vi "LVClass_WavefrontCorrector Get Actuator Current Position.vi"(0 "WavefrontCorrector in":refnum<class "WavefrontCorrector.lvclass">, 5 "Index of actuator":i32, 11 "error in (no error)":errorcluster) -> (4 "WavefrontCorrector out":refnum<class "WavefrontCorrector.lvclass">, 6 "Position":i32, 15 "error out":errorcluster)   [LabVIEW 2020, in "WavefrontCorrector.lvclass"]
doc: "Get current position of actuator.\n\n<B>correctorIn</B> : WavefrontCorrector object.\n<B>correctorOut</B> : WavefrontCorrector object.\n<B>actuator_index</B> : Index of the actuator.\n<B>position</B> : Position of the actuator."
uses:
  WavefrontCorrector.lvclass
  WavefrontCorrector.lvclass/WavefrontCorrector.ctl
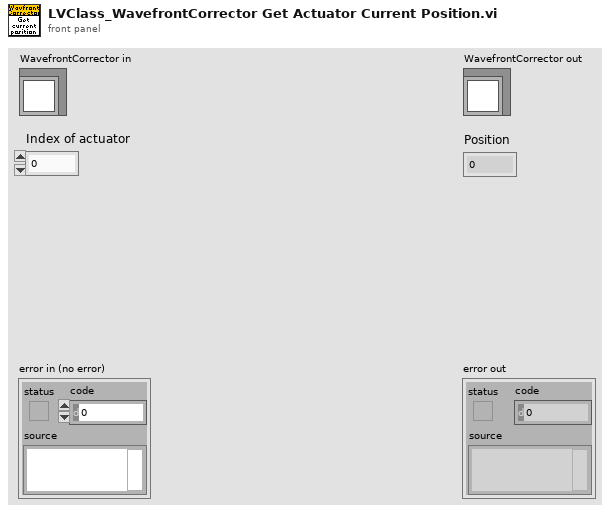
[diagram p1: front panel]
types:
  T1 = typedef "ClassID.ctl" = i64
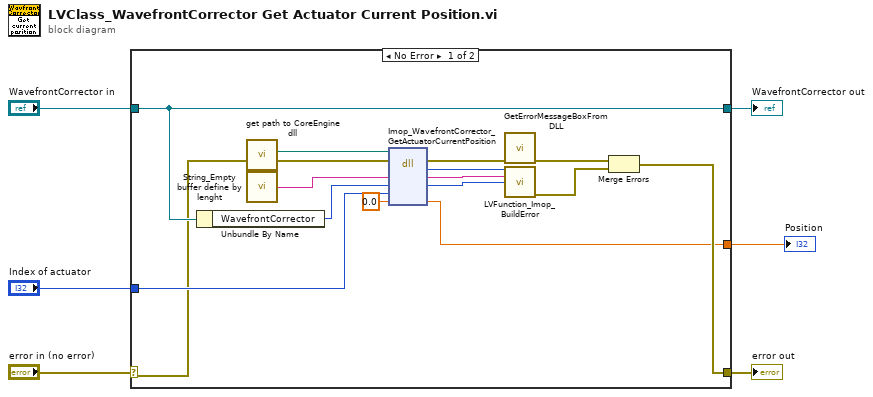
[diagram p0: block diagram]
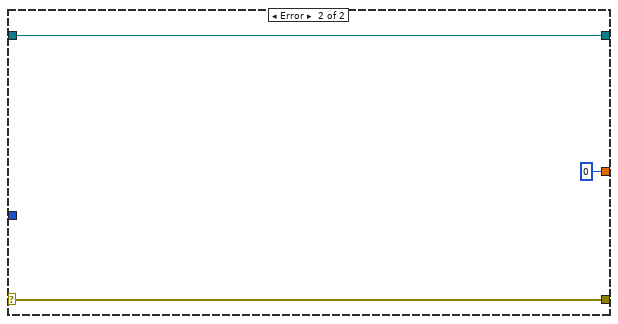
[diagram p2: hidden frame]
diagram:
  n1 = case shown="No Error" "error in (no error)" {
    selector: "error in (no error)" -> [w10 w24]
    tunnel: [w11 w24] -> w5
    tunnel: [w19 w23] -> w3
    tunnel: "WavefrontCorrector in" -> [w19 w23]
    tunnel: "Index of actuator" -> [w17 _]
    tunnel: [w9 0 ("Position")] -> w1
    frame No Error {
      n2 = Unbundle By Name(w19) -> ("WavefrontCorrector"=w18:T1)
      n3 = call "get path to CoreEngine dll.vi"() -> ("path to wavekit library"=w21:path)  [unwired: 14 in, 1 out]
      n4 = call "String_Empty buffer define by lenght.vi"() -> ("Empty buffer"=w20:string)  [unwired: 1 in]
      n5 = dll-call lib="D:/FLE/0.Code/CoreEngine4_Suite/LV2011_interface/DLLs/c_interface_vc100.dll" fn="Imop_WavefrontCorrector_GetActuatorCurrentPosition"(path in=w21, error in=w10, "Message"=w20, "WavefrontCorrector"=w18, "Index of actuator"=w17, "Position"=sgl 0.0) -> (error out=w16:errorcluster, "return type"=w14:i32, "Message"=w13:string, "WavefrontCorrector"=w7:i64, "Position"=w9:sgl)  [unwired: 2 in, 1 out]
      n6 = call "GetErrorMessageBoxFromDLL.vi"("error IN"=w16) -> ("error OUT"=w15:errorcluster)  [unwired: 10 in]
      n7 = call "LVFunction_Imop_BuildError.vi"("code"=w14, "String to Prepend to source (\"\")"=w13, "Adresse"=w7) -> ("error out"=w12:errorcluster)  [unwired: 12 in]
      n8 = Merge Errors(w15, w12) -> (w11:errorcluster)
    }
    frame Error {
    }
  }
  "error out" <- w5
  "WavefrontCorrector out" <- w3
  "Position" <- w1
